vi "open.vi"(8 "error in":errorcluster, 11 "toml file path":path) -> (0 "error out":errorcluster, 3 "toml out":refnum<class "toml.lvclass">)   [LabVIEW 2020, in "toml.lvclass"]
uses:
  toml.lvclass
  toml.lvclass/toml.ctl
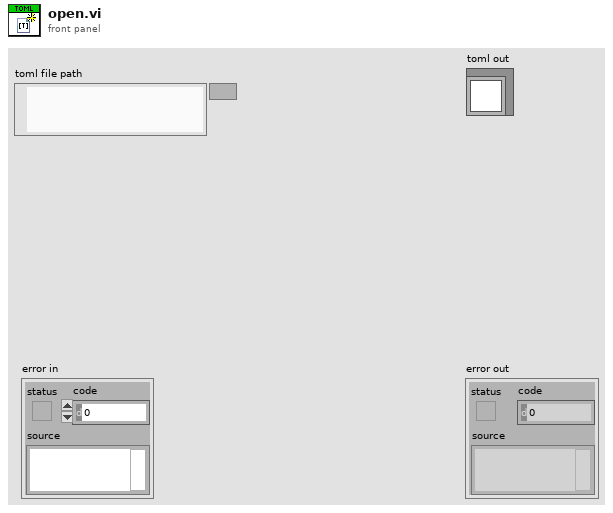
[diagram p1: front panel]
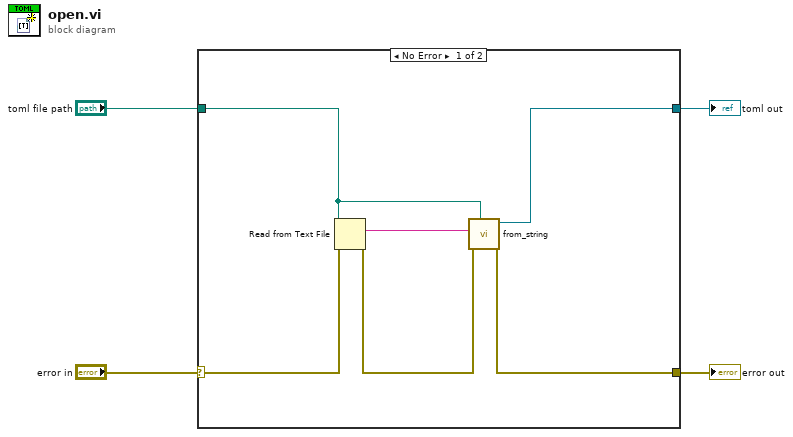
[diagram p0: block diagram]
diagram:
  n1 = case shown="No Error" "error in" {
    selector: "error in" -> [w10 w11]
    tunnel: [w6 w11] -> w3
    tunnel: [w7 _] -> w1
    tunnel: "toml file path" -> [w5 _]
    frame No Error {
      n2 = Read from Text File(file (use dialog)=w5, error in=w10) -> (text=w9:string, error out=w8:errorcluster)  [unwired: 2 in, 2 out]
      n3 = call "from_string.vi"("optional file path (to include in parse error message)"=w5, "error in (no error)"=w8, "toml"=w9) -> ("error out"=w6:errorcluster, "toml out"=w7:refnum<class "toml.lvclass">)  [unwired: 7 in]
    }
    frame Error {
    }
  }
  "error out" <- w3
  "toml out" <- w1
